vi "MsgToNestedDecorator.vi"(8 "Alias":string, 9 "Priority Msg?":bool, 10 "Msg":refnum<class "Msg Strategy.lvclass">, 11 "Dev Actor in":refnum<class "Dev Actor.lvclass">) -> (0 "error out":errorcluster)   [LabVIEW 2021, in "Dev Actor.lvlib" / "Dev Actor.lvclass"]
uses:
  Dev Actor.lvclass
  LVCAM/LVCAM/Msg Strategy/Msg Strategy.lvclass
  Dev Actor.lvclass/Dev Actor.ctl
  LVCAM/LVCAM/Actor/Actor.lvclass
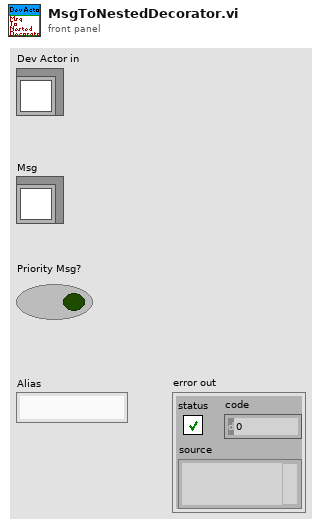
[diagram p1: front panel]
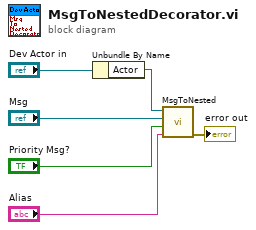
[diagram p0: block diagram]
diagram:
  n1 = Unbundle By Name("Dev Actor in") -> ("Actor"=w5:refnum<class "Actor.lvclass">)
  n2 = call-dynamic "MsgToNested.vi"("Alias"="Alias", "Priority Msg?"="Priority Msg?", "Msg"="Msg", "Actor in"=w5) -> ("error out"=→"error out":errorcluster)  [unwired: 7 in]
